vi "Teleop.vi"(10 "Match Info":T1={"Autonomous Elapsed Seconds"=0.0, "TeleOp Elapsed Seconds"=0.0, "Disabled Elapsed Seconds"=0.0, "Visited Autonomous"=FALSE, "Visited TeleOp"=FALSE, "Visited Disabled"=FALSE, "Autonomous Settings"={"Autonomous Style"=enum."Independent", "VI Refnum"=refnum}}, 11 "Call Context":T2) -> ()   [LabVIEW 2023]
doc: "This VI is called for each TeleOp packet received from the DS where the robot is not disabled. It is often used to read from the joysticks and update I/O or to update setpoints for timed control loops. It should complete and return within 20 milliseconds or it may miss DS packets."
uses:
  <vilib>/Rock Robotics/WPI/DriverStation/WPI_DriverStationDerivedRobotMode.ctl
  <vilib>/Rock Robotics/WPI/DriverStation/WPI_DriverStationMatch Info.ctl
  Global INIT.vi
  <vilib>/Rock Robotics/Network Tables/NT Read Number.vi
panel:
  out "Sample Slider 0":dbl(slide) scale=0.0..5.0
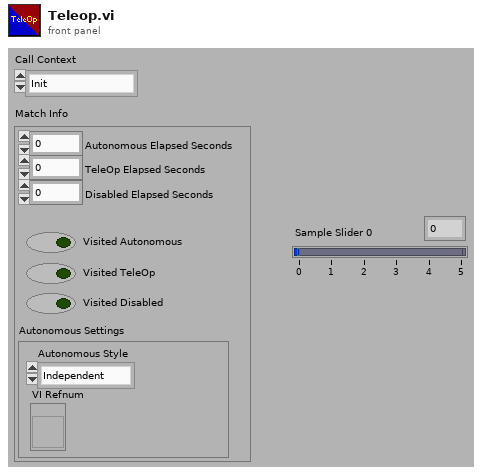
[diagram p1: front panel]
types:
  T1 = typedef "WPI_DriverStationMatch Info.ctl" = cluster{"Autonomous Elapsed Seconds":dbl, "TeleOp Elapsed Seconds":dbl, "Disabled Elapsed Seconds":dbl, "Visited Autonomous":bool, "Visited TeleOp":bool, "Visited Disabled":bool, "Autonomous Settings":cluster{"Autonomous Style":enum16{"Iterative", "Independent"}, "VI Refnum":refnum<vi>}}
  T2 = typedef "WPI_DriverStationDerivedRobotMode.ctl" = enum16{"Init", "Execute", "Stop"}
  T3 = typedef "ctrl controllers.ctl" = cluster{"Axes":dbl[], "Buttons":bool[], "POVs":i16[]}
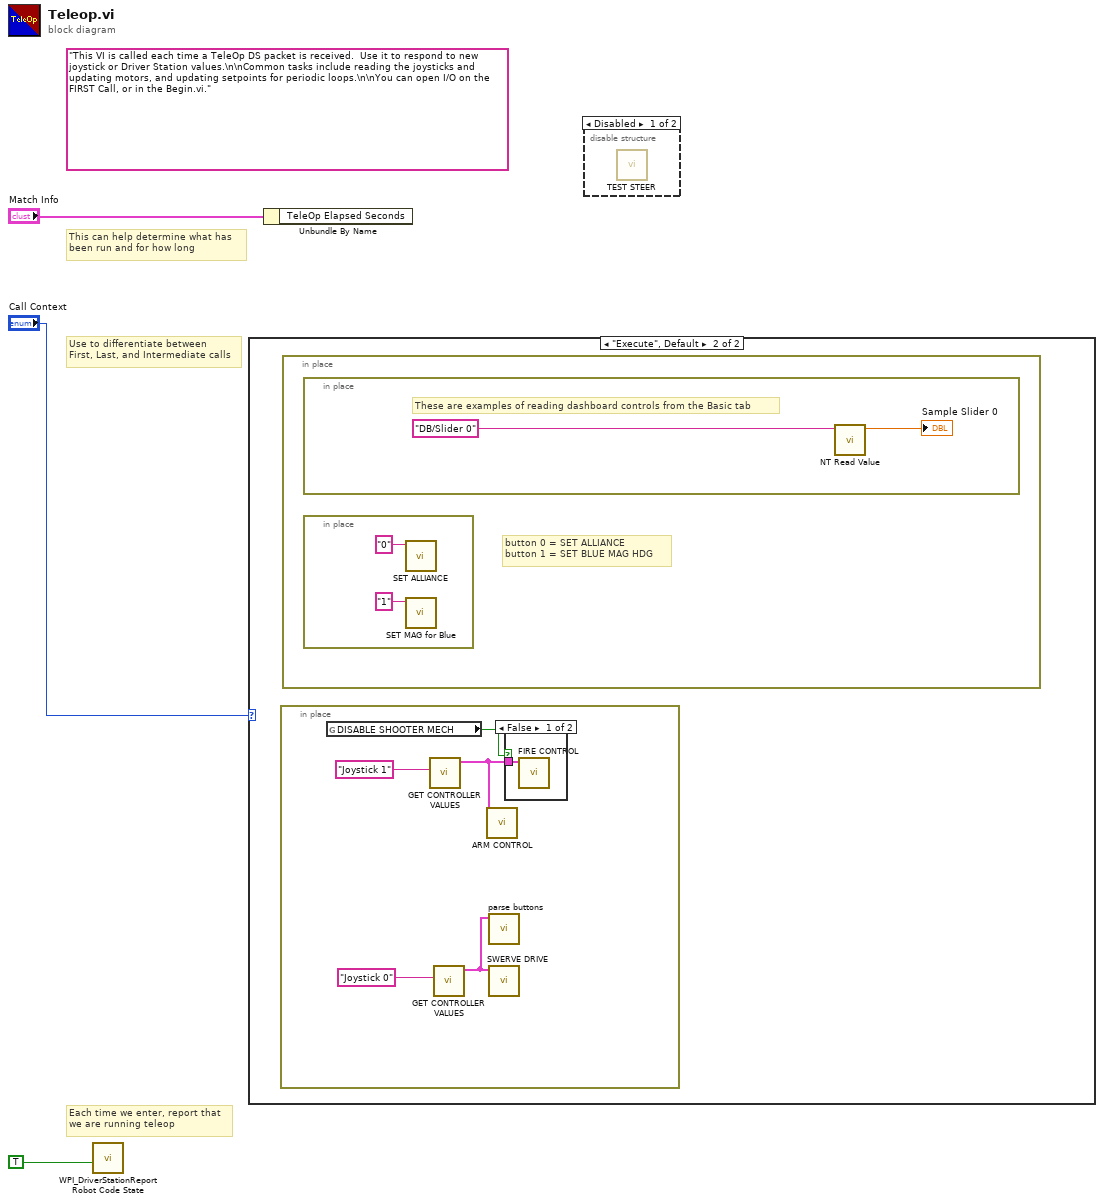
[diagram p0: block diagram]
diagram:
  (unwired) "This VI is called each time a TeleOp DS packet is received.  Use it to respond to new joystick or Driver Station values.\n\nCommon tasks include reading the joysticks and updating motors, and updating setpoints for periodic loops.\n\nYou can open I/O on the FIRST Call, or in the Begin.vi."
  # "Use to differentiate between\nFirst, Last, and Intermediate calls"
  # "Each time we enter, report that\nwe are running teleop"
  # "This can help determine what has\nbeen run and for how long"
  n1 = call <vilib>:"WPI_DriverStationReport Robot Code State.vi"("TeleOp"=TRUE ("Autonomous")) -> ()  [unwired: 10 in, 1 out]
  n2 = case shown="\"Execute\", Default" "Call Context" {
    frame "Init" {
    }
    frame "Execute", Default {
      n3 = in-place {
        n4 = global read "Global INIT.vi" "DISABLE SHOOTER MECH"() -> (w8:bool)
        n5 = call "GET CONTROLLER VALUES.vi"("controller\nrefnum name"="Joystick 1" ("refnum name")) -> ("controller out"=w9:T3)  [unwired: 9 in, 1 out]
        n6 = call "GET CONTROLLER VALUES.vi"("controller\nrefnum name"="Joystick 0" ("refnum name")) -> ("controller out"=w12:T3)  [unwired: 9 in, 1 out]
        n7 = call "ARM CONTROL.vi"("control\ncluster"=w9) -> ()  [unwired: 9 in, 2 out]
        n8 = call "parse buttons.vi"("control\ncluster"=w12) -> ()  [unwired: 9 in, 2 out]
        n9 = call "SWERVE DRIVE.vi"("controller in"=w12) -> ()  [unwired: 9 in, 2 out]
        n10 = case shown="False" w8 {
          tunnel: w9 -> [w13 _]
          frame False {
            n11 = call "FIRE CONTROL.vi"("control\ncluster"=w13) -> ()  [unwired: 9 in, 2 out]
          }
          frame True {
          }
        }
      }
      n12 = in-place {
        # "button 0 = SET ALLIANCE\nbutton 1 = SET BLUE MAG HDG"
        n13 = in-place {
          # "These are examples of reading dashboard controls from the Basic tab"
          n14 = call-poly <vilib>:"NT Read Value.vi"("name"="DB/Slider 0" ("refnum name")) -> ("value"=→"Sample Slider 0":dbl)  [unwired: 8 in, 2 out]
        }
        n15 = in-place {
          n16 = call "SET ALLIANCE.vi"("stack name"="0" ("refnum name")) -> ()  [unwired: 9 in, 2 out]
          n17 = call "SET MAG for Blue.vi"("stack name"="1" ("refnum name")) -> ()  [unwired: 9 in, 2 out]
        }
      }
    }
  }
  n18 = Unbundle By Name("Match Info") -> ()  [unwired: 1 out]
  n19 = disable-structure shown="Disabled" {
    frame Disabled {
      n20 = call "TEST STEER.vi"() -> ()  [unwired: 12 in]
    }
    frame Enabled {
    }
  }
